vi "PS Control Read.vi"(5 "error in":errorcluster, 6 "Read State":T1(ring)=enum."Read-Status", 8 "Magnet System":enum16{"Resistive", "Hybrid"}(ring)) -> (0 "error out":errorcluster, 1 "Cell":string, 2 "Current Field":dbl caption="Current [T]" format="%.5f", 3 "Status":T2, 4 "Current Setpoint (T)":dbl caption="Current Setpoint" format="%.5f")   [LabVIEW 2020]
panel:
  out "Time(ms)":u32
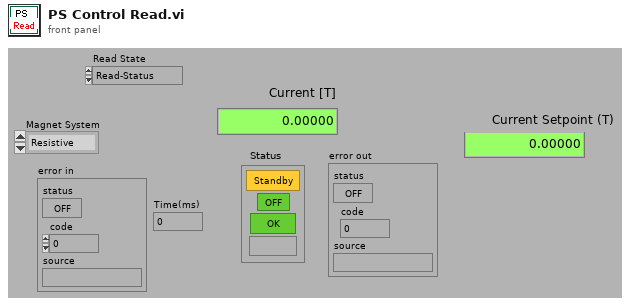
[diagram p1: front panel]
types:
  T1 = enum16{"--Quit--", "Read-Status", "Read-Cell", "Read-Field[T]", "Read-Setpoint[T]"}
  T2 = cluster{"PS on/off":bool, "PS fault?":bool, "Ramp Status":u16, "PS Control?":bool}
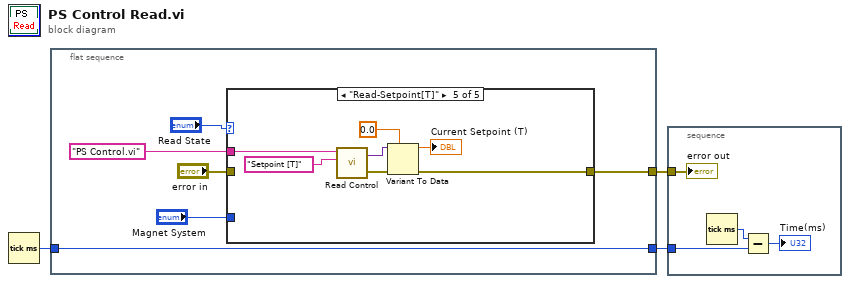
[diagram p0: block diagram]
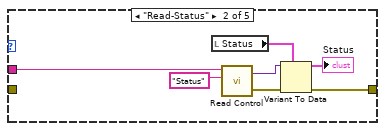
[diagram p3: hidden frame]
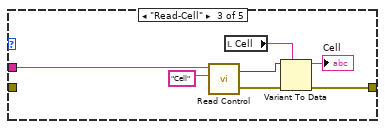
[diagram p4: hidden frame]
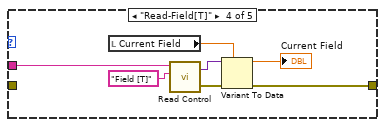
[diagram p5: hidden frame]
diagram:
  n1 = Tick Count (ms)() -> (millisecond timer value=w2:u32)
  n2 = flat-sequence {
    tunnel: [w4] -> w3
    tunnel: w2 -> [w7]
    tunnel: [w7] -> w1
    frame #0 {
      n3 = case shown="\"Read-Setpoint[T]\"" "Read State" {
        tunnel: "error in" -> [w10 _ _ _ _]
        tunnel: [w10 w16 w20 w29 w36] -> w4
        tunnel: "Magnet System" -> [_ _ _ _ _]
        tunnel: "PS Control.vi" -> [_ w15 w22 w26 w33]
        frame "--Quit--", Default {
        }
        frame "Read-Status" {
          n4 = local read "Status"() -> (w12:T2)
          n5 = call "Read Control.vi"("VI Name"=w15, "Control Name"="Status") -> ("Value"=w13:variant, "error out"=w11:errorcluster)  [unwired: 3 in]
          n6 = Variant To Data(error in=w11, type=w12, Variant=w13) -> (data=→"Status":T2, error out=w16:errorcluster)
        }
        frame "Read-Cell" {
          n7 = call "Read Control.vi"("VI Name"=w22, "Control Name"="Cell") -> ("Value"=w24:variant, "error out"=w23:errorcluster)  [unwired: 3 in]
          n8 = local read "Cell"() -> (w18:string)
          n9 = Variant To Data(error in=w23, type=w18, Variant=w24) -> (data=→"Cell":string, error out=w20:errorcluster)
        }
        frame "Read-Field[T]" {
          n10 = local read "Current Field"() -> (w27:dbl)
          n11 = call "Read Control.vi"("VI Name"=w26, "Control Name"="Field [T]") -> ("Value"=w31:variant, "error out"=w30:errorcluster)  [unwired: 3 in]
          n12 = Variant To Data(error in=w30, type=w27, Variant=w31) -> (data=→"Current Field":dbl, error out=w29:errorcluster)
        }
        frame "Read-Setpoint[T]" {
          n13 = call "Read Control.vi"("VI Name"=w33, "Control Name"="Setpoint [T]") -> ("Value"=w38:variant, "error out"=w37:errorcluster)  [unwired: 3 in]
          n14 = Variant To Data(error in=w37, type=0.0 ("Current Setpoint (T)"), Variant=w38) -> (data=→"Current Setpoint (T)":dbl, error out=w36:errorcluster)
        }
      }
    }
  }
  n15 = stacked-sequence {
    tunnel: w1 -> [w41]
    tunnel: w3 -> [w39]
    frame #0 {
      n16 = Tick Count (ms)() -> (millisecond timer value=w42:u32)
      n17 = Subtract(x=w42, y=w41) -> (x-y=→"Time(ms)":u32)
      "error out" <- w39
    }
  }
